vi "getGrating.vi"(8 "error in (no error)":errorcluster, 11 "Monochromator in":refnum<class "Monochromator.lvclass">) -> (0 "error out":errorcluster, 2 "GratingType":T1=enum."Red", 3 "Monochromator out":refnum<class "Monochromator.lvclass">)   [LabVIEW 2016, in "Monochromator.lvclass"]
uses:
  Monochromator.lvclass
  Typedefs/GratingType.ctl
  Monochromator.lvclass/Monochromator.ctl
  MonoStates/MonoState/MonoState.lvclass
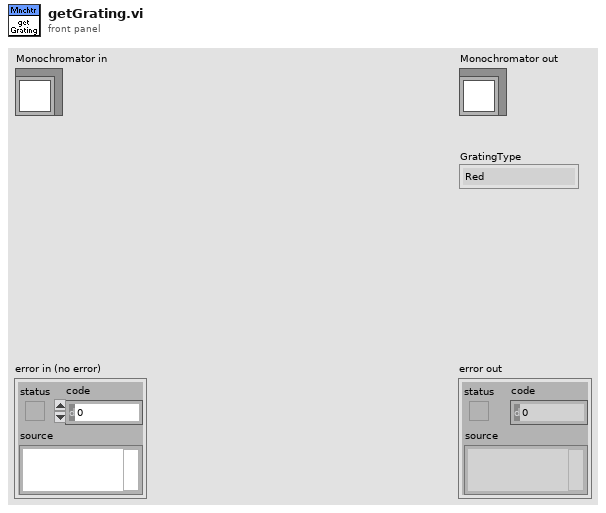
[diagram p1: front panel]
types:
  T1 = typedef "GratingType.ctl" = enum16{"NoGrating", "Red", "Blue", "Mirror"}
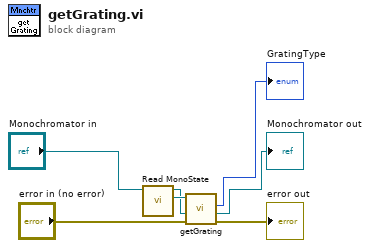
[diagram p0: block diagram]
diagram:
  n1 = call "Read MonoState.vi"("Monochromator in"="Monochromator in") -> ("MonoState.lvclass"=w2:refnum<class "MonoState.lvclass">, "Monochromator out"=w1:refnum<class "Monochromator.lvclass">)  [unwired: 8 in, 1 out]
  n2 = call-dynamic "getGrating.vi"("error in (no error)"="error in (no error)", "Monochromator in"=w1, "MonoState in"=w2) -> ("error out"=→"error out":errorcluster, "Monochromator out"=→"Monochromator out":refnum<class "Monochromator.lvclass">, "GratingType"=→"GratingType":T1)  [unwired: 5 in, 1 out]
